vi "TwTpsGetStatus.vi"(7 "error in (no error)":errorcluster) -> (0 "ion mode":string, 1 "canChangeIonMode?":bool, 2 "changeIonModeSupported?":bool, 3 "error out":errorcluster, 4 "shutdown?":bool, 5 "initialized?":bool, 6 "connected?":bool)   [LabVIEW 2009]
uses:
  TofDaqDll.dll
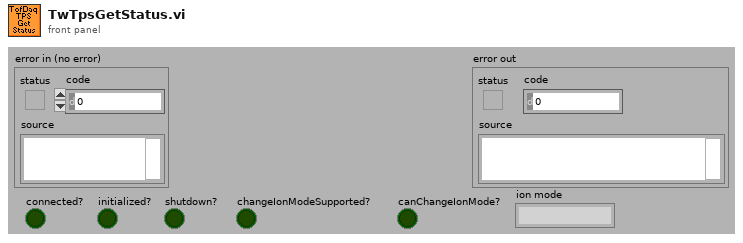
[diagram p1: front panel]
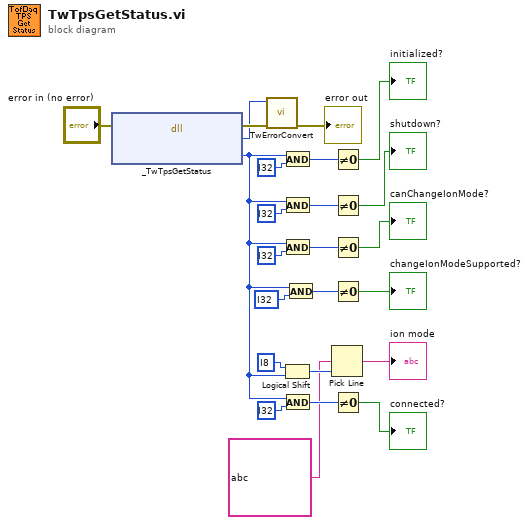
[diagram p0: block diagram]
diagram:
  n1 = dll-call lib="C:/src/TofDaq/APIandWrappers/LabView/TofDaqDll/TofDaqDll.dll" fn="_TwTpsGetStatus"(error in="error in (no error)") -> (error out=w23:errorcluster, "TwRetVal"=w21:i32, "status"=w5:i32)  [unwired: 2 in, 2 out]
  n2 = call "TwErrorConvert.vi"("error in (no error)"=w23, "error code"=w21) -> ("error out"=→"error out":errorcluster)  [unwired: 9 out]
  n3 = Logical Shift(y=i8 ?, x=w5) -> (x << y=w3:i32)
  n4 = And(x=w5, y=i32 ?) -> (x .and. y?=w16:i32)
  n5 = And(x=w5, y=i32 ?) -> (x .and. y?=w13:i32)
  n6 = And(x=w5, y=i32 ?) -> (x .and. y?=w10:i32)
  n7 = And(x=w5, y=i32 ?) -> (x .and. y?=w19:i32)
  n8 = And(x=w5, y=i32 ?) -> (x .and. y?=w7:i32)
  n9 = Pick Line(multi-line string=string ?, line index=w3) -> (output string=→"ion mode":string)  [unwired: 1 in]
  n10 = Not Equal To 0?(x=w16) -> (x != 0?=→"initialized?":bool)
  n11 = Not Equal To 0?(x=w13) -> (x != 0?=→"shutdown?":bool)
  n12 = Not Equal To 0?(x=w10) -> (x != 0?=→"canChangeIonMode?":bool)
  n13 = Not Equal To 0?(x=w7) -> (x != 0?=→"changeIonModeSupported?":bool)
  n14 = Not Equal To 0?(x=w19) -> (x != 0?=→"connected?":bool)
